vi "PFI-28000-Chan-28144_Get Expected Loop Resistance.vi"(8 "error in (no error)":errorcluster, 11 "PFI-28000-Chan-28144 in":refnum<class "PFI-28000-Chan-28144.lvclass">) -> (0 "error out":errorcluster, 2 "Expected Loop Resistance":dbl, 3 "PFI-28000-Chan-28144 out":refnum<class "PFI-28000-Chan-28144.lvclass">)   [LabVIEW 2017, in "PFI-28000-Chan-28144.lvclass"]
uses:
  PFI-28000-Chan-28144.lvclass
  C:/wc/07143 Precision Filters 28000 Support/Driver/source/Channel/PFI-28000-Channel.lvclass
  Utilities/PFI-28000-Utils.lvlib
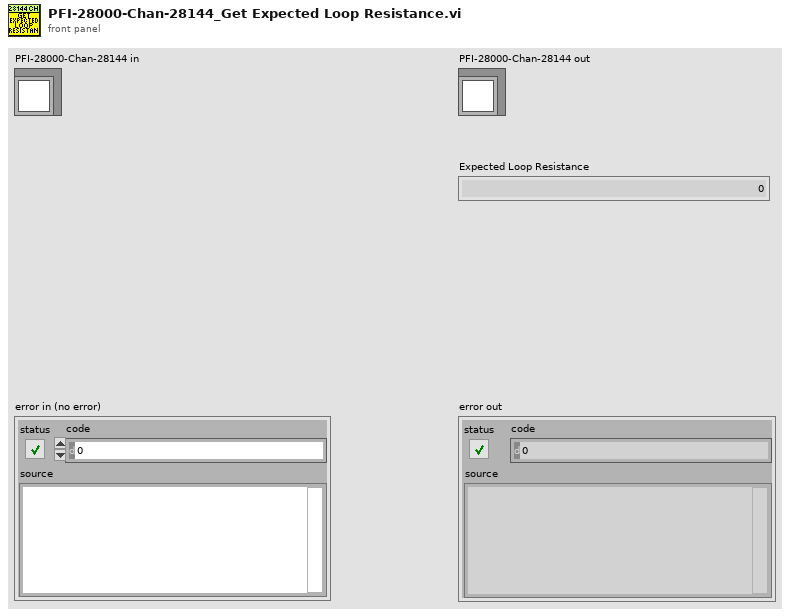
[diagram p1: front panel]
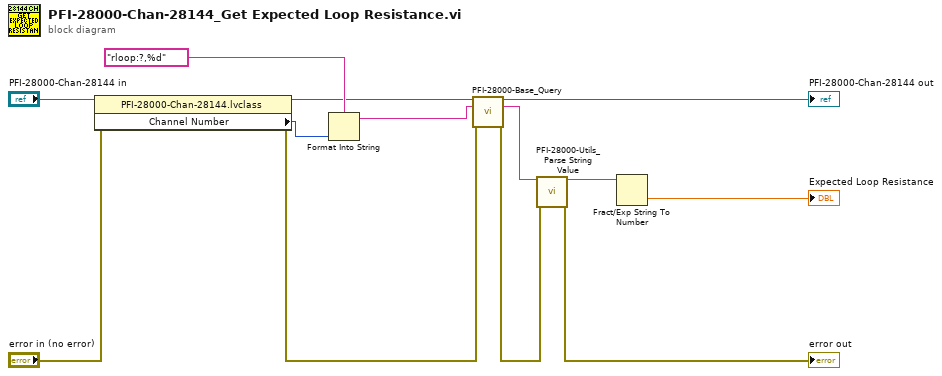
[diagram p0: block diagram]
diagram:
  n1 = property class="PFI-28000-Chan-28144.lvclass"(reference="PFI-28000-Chan-28144 in", error in="error in (no error)") -> (reference out=w9:refnum<class "PFI-28000-Chan-28144.lvclass">, error out=w7:errorcluster, "Channel Number"=w11:i32)
  n2 = Format Into String(format string="rloop:?,%d" ("empty string"), w11) -> (resulting string=w8:string)  [unwired: 2 in, 1 out]
  n3 = call-dynamic "PFI-28000-Base_Query.vi"("PFI-28000-Base in"=w9, "Command"=w8, "error in (no error)"=w7) -> ("PFI-28000-Base out"=→"PFI-28000-Chan-28144 out":refnum<class "PFI-28000-Chan-28144.lvclass">, "Response"=w4:string, "error out"=w2:errorcluster)  [unwired: 9 in, 1 out]
  n4 = call "PFI-28000-Utils_Parse String Value.vi"("String"=w4, "error in (no error)"=w2) -> ("String Value"=w3:string, "error out"=→"error out":errorcluster)  [unwired: 11 in, 1 out]
  n5 = Fract/Exp String To Number(string=w3) -> (number=→"Expected Loop Resistance":dbl)  [unwired: 3 in, 1 out]
